vi "Teleop_Out_Lifter.vi"(8 "error in (no error)":errorcluster, 11 "Teleop Local Data Out":T1) -> (0 "error out":errorcluster)   [LabVIEW 2016]
uses:
  Typedefs/typedef_cluster_Teleop Local Data.ctl
  <vilib>/Rock Robotics/WPI/Solenoid/WPI_SolenoidValue.ctl
  <vilib>/Rock Robotics/WPI/Solenoid/WPI_SolenoidSetEnum.vi
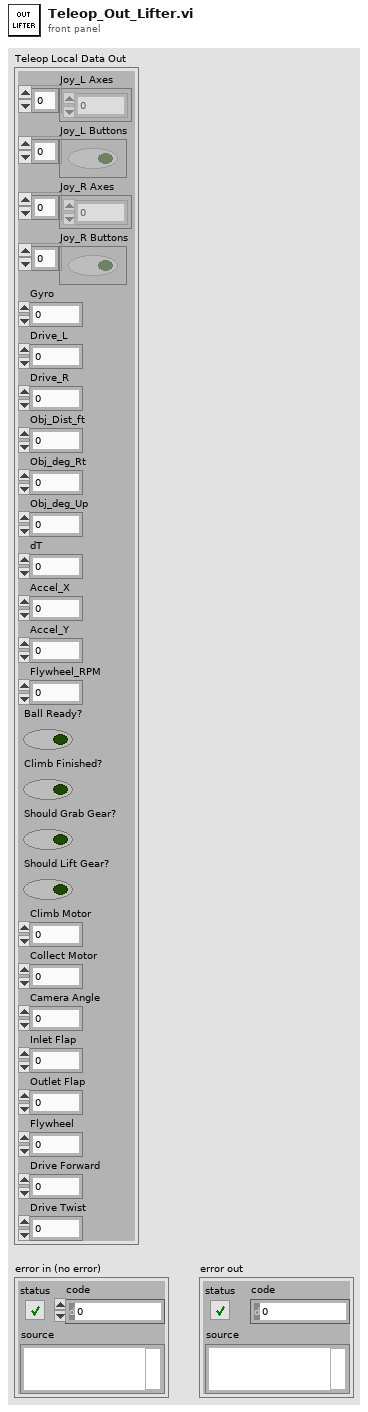
[diagram p1: front panel]
types:
  T1 = typedef "typedef_cluster_Teleop Local Data.ctl" = cluster{"Joy_L Axes":dbl[], "Joy_L Buttons":bool[], "Joy_R Axes":dbl[], "Joy_R Buttons":bool[], "Gyro":dbl, "Drive_L":i32, "Drive_R":i32, "Obj_Dist_ft":dbl, "Obj_deg_Rt":dbl, "Obj_deg_Up":dbl, "dT":dbl, "Accel_X":dbl, "Accel_Y":dbl, "Flywheel_RPM":dbl, "Ball Ready?":bool, "Climb Finished?":bool, "Should Grab Gear?":bool, "Should Lift Gear?":bool, "Climb Motor":dbl, "Collect Motor":dbl, "Camera Angle":dbl, "Inlet Flap":dbl, "Outlet Flap":dbl, "Flywheel":dbl, "Drive Forward":dbl, "Drive Twist":dbl}
  T2 = typedef "WPI_SolenoidValue.ctl" = enum16{"Off", "On", "Forward", "Reverse"}
  T3 = typedef "WPI_SolenoidDevRef.ctl" = cluster{"DevStatus":errorcluster, "Pneumatics Control Module":u8, "Forward Solenoid Channel":T4, "Reverse Solenoid Channel":T4}
  T4 = typedef "WPI_SolenoidChannel.ctl" = enum8{"Solenoid 0", "Solenoid 1", "Solenoid 2", "Solenoid 3", "Solenoid 4", "Solenoid 5", "Solenoid 6", "Solenoid 7", "Invalid"}
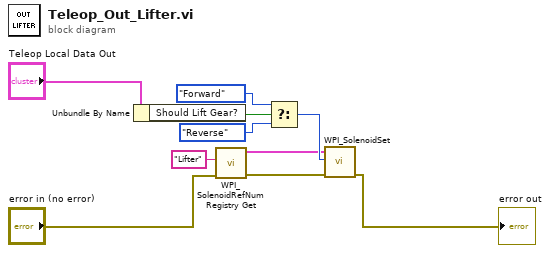
[diagram p0: block diagram]
diagram:
  n1 = Unbundle By Name("Teleop Local Data Out") -> ("Should Lift Gear?"=w4:bool)
  n2 = call <vilib>:"WPI_SolenoidRefNum Registry Get.vi"("error in (no error)"="error in (no error)", "refnum name"="Lifter") -> ("error out"=w3:errorcluster, "SolenoidDevRef"=w2:T3)  [unwired: 8 in]
  n3 = Select(t=WPI_SolenoidValue."Forward" ("Value"), s=w4, f=WPI_SolenoidValue."Reverse" ("Value")) -> (s? t:f=w5:T2)
  n4 = call-poly <vilib>:"WPI_SolenoidSet.vi"("error in (no error)"=w3, "Value"=w5, "SolenoidDevRef"=w2) -> ("error out"=→"error out":errorcluster)  [unwired: 7 in, 1 out]
